vi "Main Page.vi"(8 "error in (no error)":errorcluster, 11 "Node Ptr":T1 format="%.0x") -> (0 "error out":errorcluster)   [LabVIEW 2019, in "Protection and Counter Addon System Explorer.lvlib"]
uses:
  Protection and Counter Addon System Explorer.lvlib
  <vilib>/NI VeriStand/Custom Device API/Custom Device Item Ref.ctl
  <vilib>/NI/NI VeriStand Hardware Resource Discovery/_Types/Filter Type.ctl
  Addon Shared/Types/986x.ctl
  Addon Shared/SubVIs/GUID Lookup.vi
  <vilib>/NI VeriStand/Custom Device API/NI VeriStand - Get Item Property.vi
  <vilib>/NI VeriStand/Custom Device API/Get Item Property (Boolean).vi
  <vilib>/NI VeriStand/Custom Device API/Get Item Property (String).vi
  <vilib>/NI VeriStand/Custom Device API/Get Item Property (Dependent File).vi
  <vilib>/NI VeriStand/Custom Device API/Custom Device API.lvlib
  <vilib>/NI/NI VeriStand Hardware Resource Discovery/NIVS Hardware Discovery.lvlib
  Addon Shared/Protection and Counter Addon Shared.lvlib
panel:
  out "Version":string
  in  "FPGA Settings":cluster{"Section Name":string}={"Section Name"="FPGA Settings"}
  in  "RIO Browse":bool
  in  "RIO Device":string
  in  "Enable Bitfile":bool
  in  "Bitfile Path":path
  in  "Use Legacy":bool
  in  "Loop Priority":i32=100 format="%.0p"
  in  "FD Baud rate [Bd]":u64 format="%.0p"
  in  "CAN I/O Mode":u32(ring) items=["CAN 2.0", "CAN FD", "CAN FD+BRS"]
  in  "Database Settings":cluster{"Section Name":string}={"Section Name"="Database Settings"}
  in  "CAN Browse":bool
  in  "Termination":enum16{"Off", "On"}(ring)
  in  "CAN Port":string
  in  "Baud rate [Bd]":u64 format="%.0p"
  out "XNET Cluster":refnum<k21>
  out "XNET Database":refnum<k21>
  in  "SHDocVw.IWebBrowser2":refnum<k7>(container)
  in  "Header":cluster{"Section Name":string}={"Section Name"="CAN Settings"}
  in  "Name":string
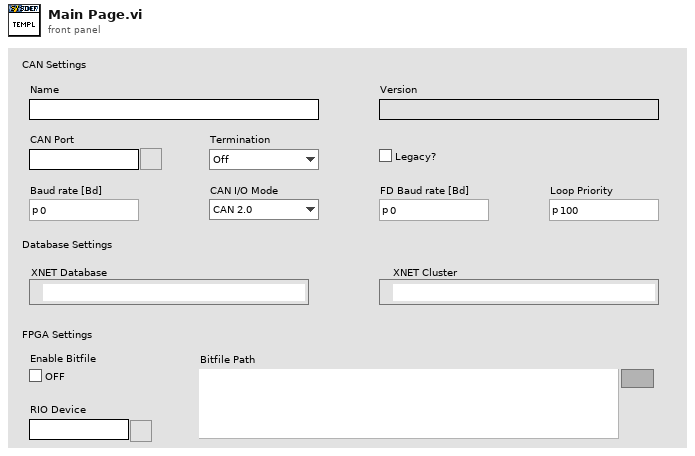
[diagram p1: front panel]
types:
  T1 = typedef "Custom Device API.lvlib/Custom Device Item Ref.ctl" = u64
  T2 = typedef "Protection and Counter Addon Shared.lvlib/986x.ctl" = cluster{"Enable":bool, "RIO Device":string, "Bitfile":path}
  T3 = typedef "Protection and Counter Addon Shared.lvlib/XNET Settings.ctl" = cluster{"Database":refnum<k21>, "Cluster":refnum<k21>, "Port":string, "Baud rate [Bd]":u64, "Termination":u32, "CAN I/O Mode":u32, "FD Baud rate [Bd]":u64, "Priority":i32, "Use Legacy":bool}
  T4 = typedef "Custom Device API.lvlib/Custom Device Item Info.ctl" = cluster{"Name":string, "Is Channel":bool, "GUID":string, "Is Waveform":bool}
  T5 = typedef "NIVS Hardware Discovery.lvlib/Filter Type.ctl" = enum16{"Device Category", "Product Name", "Ethernet", "XNET", "VISA", "FPGA", "EtherCAT Master", "DAQmx", "GPIB", "Serial"}
  T6 = typedef "Custom Device API.lvlib/Custom Device Commands.ctl" = enum16{"Default", "Item renamed", "Shutdown", "Dynamic button pressed"}
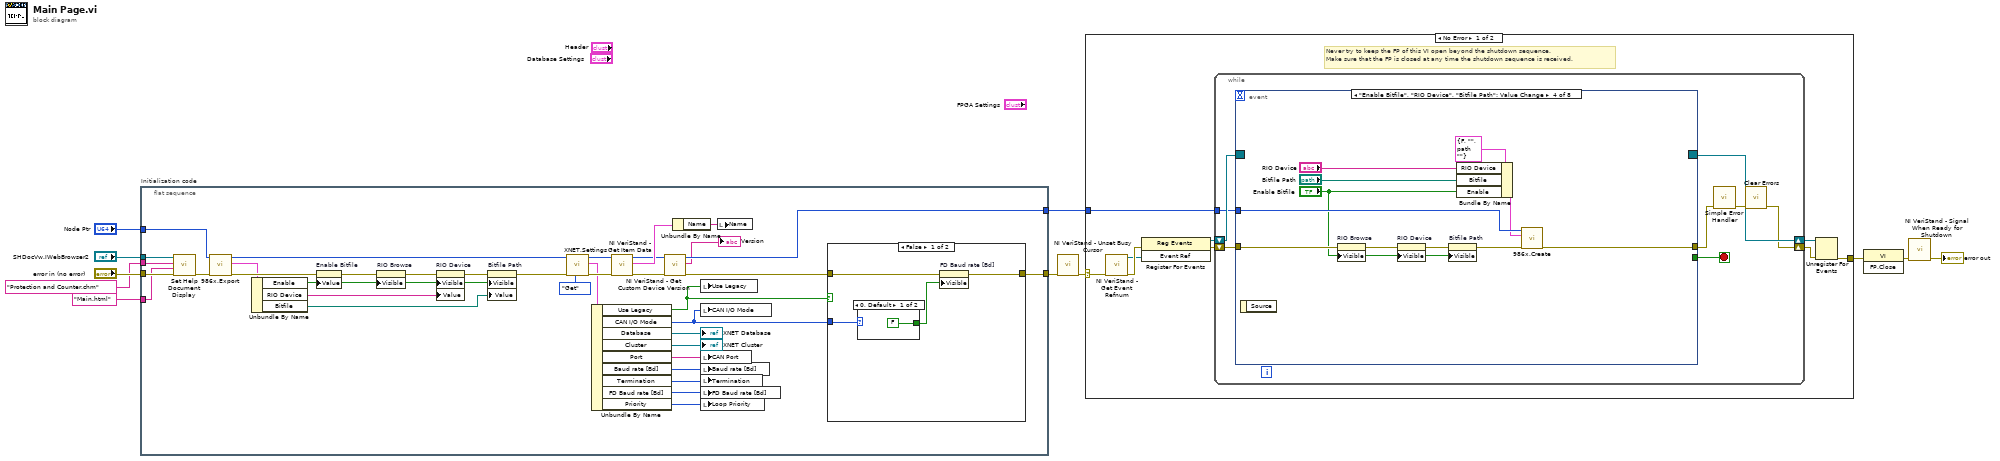
[diagram p0: block diagram]
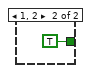
[diagram p2: hidden frame]
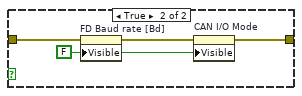
[diagram p3: hidden frame]
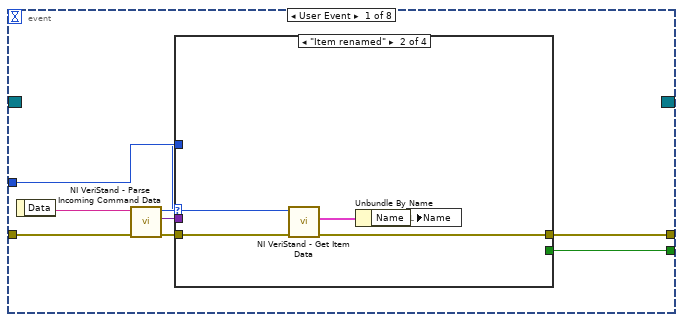
[diagram p4: hidden frame]
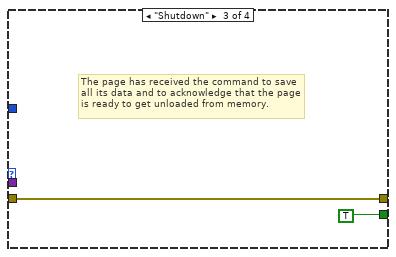
[diagram p6: hidden frame]
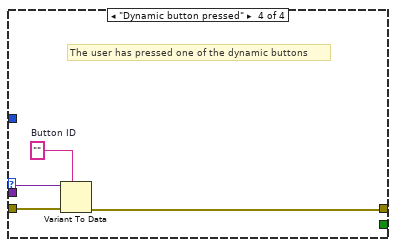
[diagram p7: hidden frame]
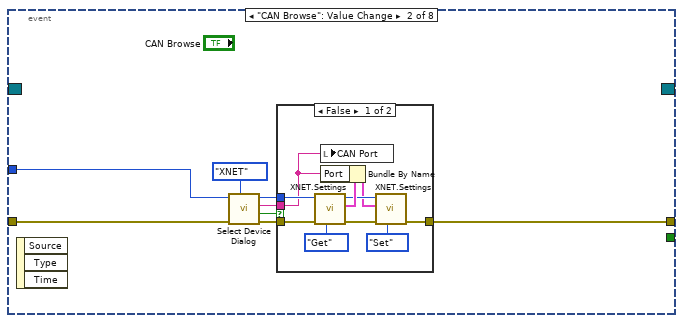
[diagram p8: hidden frame]
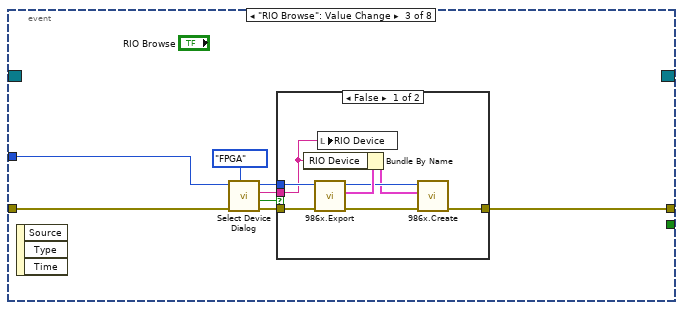
[diagram p10: hidden frame]
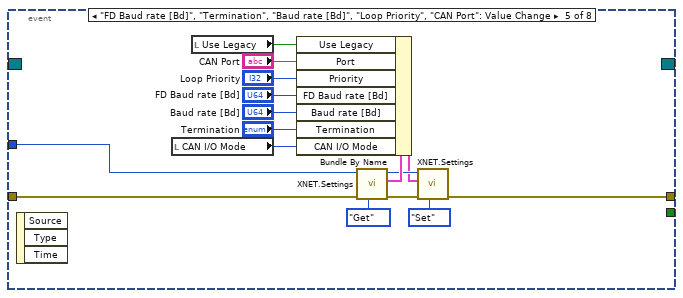
[diagram p12: hidden frame]
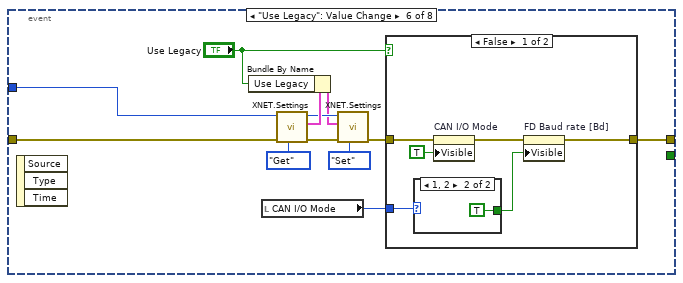
[diagram p13: hidden frame]
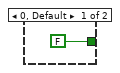
[diagram p14: hidden frame]
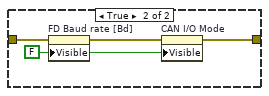
[diagram p15: hidden frame]
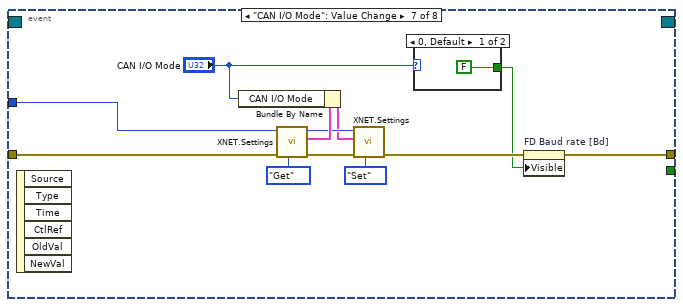
[diagram p16: hidden frame]
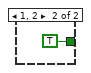
[diagram p17: hidden frame]
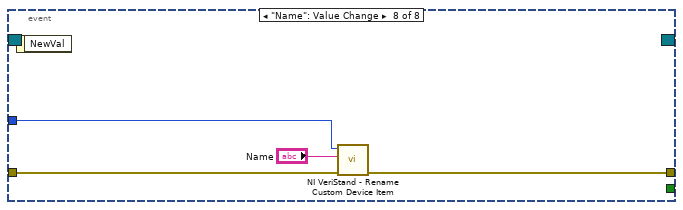
[diagram p18: hidden frame]
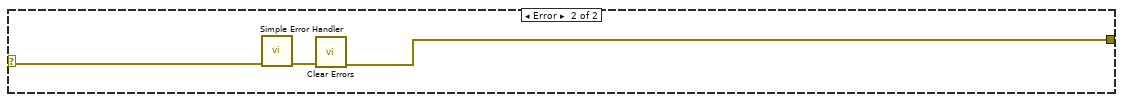
[diagram p19: hidden frame]
diagram:
  n1 = flat-sequence "Initialization code" {
    tunnel: "error in (no error)" -> [w46]
    tunnel: "Node Ptr" -> [w27]
    tunnel: [w30] -> w7
    tunnel: [w13] -> w4
    tunnel: "SHDocVw.IWebBrowser2" -> [w45]
    tunnel: "Protection and Counter.chm" ("Main CHM File") -> [w44]
    tunnel: "Main.html" ("HTML File") -> [w43]
    frame #0 {
      n2 = call "Set Help Document Display.vi"("error in (no error)"=w46, "HTML File"=w43, "Main CHM File"=w44, "SHDocVw.IWebBrowser2"=w45) -> ("error out"=w28:errorcluster)  [unwired: 7 in]
      n3 = call "986x.Export.vi"("error in (no error)"=w28, "Device Item Ref in"=w27) -> ("error out"=w22:errorcluster, "986x Support"=w20:T2, "Item Ref out"=w26:T1)  [unwired: 7 in]
      n4 = Unbundle By Name(w20) -> ("Enable"=w19:bool, "RIO Device"=w18:string, "Bitfile"=w17:path)
      n5 = property on="Enable Bitfile" class="Bool (strict)"(error in=w22, "Value"=w19) -> (error out=w25:errorcluster)  [unwired: 1 in, 1 out]
      n6 = property on="RIO Browse" class="Bool"(error in=w25, "Visible"=w19) -> (error out=w24:errorcluster)  [unwired: 1 in, 1 out]
      n7 = property on="RIO Device" class="Str"(error in=w24, "Visible"=w19, "Value"=w18) -> (error out=w23:errorcluster)  [unwired: 1 in, 1 out]
      n8 = property on="Bitfile Path" class="Path"(error in=w23, "Visible"=w19, "Value"=w17) -> (error out=w21:errorcluster)  [unwired: 1 in, 1 out]
      n9 = call "XNET.Settings.vi"("Action"=enum8{"Get", "Set"}."Get", "error in (no error)"=w21, "Parent Ref in"=w26) -> ("error out"=w42:errorcluster, "XNET Settings"=w39:T3, "Item Ref out"=w41:T1)  [unwired: 6 in]
      n10 = Unbundle By Name(w39) -> ("Use Legacy"=w31:bool, "CAN I/O Mode"=w29:u32, "Database"=→"XNET Database":refnum<k21>, "Cluster"=→"XNET Cluster":refnum<k21>, "Port"=w36:string, "Baud rate [Bd]"=w35:u64, "Termination"=w34:u32, "FD Baud rate [Bd]"=w33:u64, "Priority"=w32:i32)
      n11 = call <vilib>:"NI VeriStand - Get Item Data.vi"("error in (no error)"=w42, "Item Ref in"=w41) -> ("error out"=w16:errorcluster, "Item Info"=w48:T4, "Item Ref out"=w14:T1)  [unwired: 7 out]
      n12 = call <vilib>:"NI VeriStand - Get Custom Device Version.vi"("error in (no error)"=w16, "Device Ref in"=w14) -> ("error out"=w15:errorcluster, "Value"=→"Version":string, "Device Ref out"=w13:T1)  [unwired: 7 in]
      n13 = Unbundle By Name(w48) -> ("Name"=w47:string)
      n14 = local write "Use Legacy"(w31) -> ()
      n15 = local write "CAN I/O Mode"(w29) -> ()
      n16 = local write "CAN Port"(w36) -> ()
      n17 = local write "Baud rate [Bd]"(w35) -> ()
      n18 = local write "Termination"(w34) -> ()
      n19 = local write "FD Baud rate [Bd]"(w33) -> ()
      n20 = local write "Loop Priority"(w32) -> ()
      n21 = local write "Name"(w47) -> ()
      n22 = case shown="False" w31 {
        tunnel: w15 -> [w51 w57]
        tunnel: [w50 w56] -> w30
        tunnel: w29 -> [w52 _]
        frame False {
          n23 = case shown="0, Default" w52 {
            tunnel: [FALSE TRUE] -> w49
            frame 0, Default {
            }
            frame 1, 2 {
            }
          }
          n24 = property on="FD Baud rate [Bd]" class="DigNum (strict)"(error in=w51, "Visible"=w49) -> (error out=w50:errorcluster)  [unwired: 1 in, 1 out]
        }
        frame True {
          w55 = FALSE ("Visible")
          n25 = property on="FD Baud rate [Bd]" class="DigNum (strict)"(error in=w57, "Visible"=w55) -> (error out=w58:errorcluster)  [unwired: 1 in, 1 out]
          n26 = property on="CAN I/O Mode" class="Ring (strict)"(error in=w58, "Visible"=w55) -> (error out=w56:errorcluster)  [unwired: 1 in, 1 out]
        }
      }
    }
  }
  n27 = call <vilib>:"NI VeriStand - Unset Busy Cursor.vi"("error in (no error)"=w7) -> ("error out"=w6:errorcluster)  [unwired: 10 out]
  n28 = case shown="No Error" w6 {
    selector: w6 -> [w59 w203]
    tunnel: [w64 w201] -> w11
    tunnel: w4 -> [w60 _]
    frame No Error {
      # "Never try to keep the FP of this VI open beyond the shutdown sequence.\nMake sure that the FP is closed at any time the shutdown sequence is received."
      n29 = call <vilib>:"NI VeriStand - Get Event Refnum.vi"("error in (no error)"=w59) -> ("error out"=w67:errorcluster, "Event Ref"=w63:refnum<user-event>)  [unwired: 9 out]
      n30 = register-events(error in=w67, w63) -> (reference out=w61:refnum<event-registration>, error out=w62:errorcluster)  [unwired: 1 in]
      n31 = while {
        tunnel: w60 -> [w71]
        shift-right: [w68] -> w65
        shift-left: w62 -> [w74]
        shift-right: [w75] -> w66
        shift-left: w61 -> [w73]
        stop <- w72 stop-if-true
        n32 = event shown="[3] \"Enable Bitfile\", \"RIO Device\", \"Bitfile Path\": Value Change" {
          selector: w73 -> [_ _ _ _ _ _ _ _]
          dyn-events: [_ _ _ _ _ _ _ _] -> w75
          timeout: _ -> [_ _ _ _ _ _ _ _]
          tunnel: w74 -> [w83 w98 w117 w139 w152 w164 w188 w200]
          tunnel: [w79 _ _ _ _ _ _ _] -> w72
          tunnel: [w78 w96 w115 w142 w151 w160 w185 w199] -> w70
          tunnel: w71 -> [w77 w97 w116 w137 w150 w163 w187 w198]
          event User Event {
            n33 = event-data() -> ("Data"=w82:string)  [unwired: 1 out]
            n34 = call <vilib>:"NI VeriStand - Parse Incoming Command Data.vi"("error in (no error)"=w83, "Incoming data"=w82) -> ("error out"=w81:errorcluster, "Outgoing data"=w76:variant, "Action"=w80:T6)  [unwired: 7 out]
            n35 = case shown="\"Item renamed\"" w80 {
              tunnel: w81 -> [w84 w89 w90 w95]
              tunnel: [_ _ TRUE _] -> w79
              tunnel: [w84 w86 w90 w92] -> w78
              tunnel: w77 -> [_ w88 _ _]
              tunnel: w76 -> [_ _ _ w94]
              frame "Default", Default {
              }
              frame "Item renamed" {
                n36 = call <vilib>:"NI VeriStand - Get Item Data.vi"("error in (no error)"=w89, "Item Ref in"=w88) -> ("error out"=w86:errorcluster, "Item Info"=w87:T4)  [unwired: 8 out]
                n37 = Unbundle By Name(w87) -> ("Name"=w85:string)
                n38 = local write "Name"(w85) -> ()
              }
              frame "Shutdown" {
                # "The page has received the command to save all its data and to acknowledge that the page is ready to get unloaded from memory."
              }
              frame "Dynamic button pressed" {
                w93 = ""  # Button ID
                # "The user has pressed one of the dynamic buttons"
                n39 = Variant To Data(error in=w95, type=w93, Variant=w94) -> (error out=w92:errorcluster)  [unwired: 1 out]
              }
            }
          }
          event "CAN Browse": Value Change {
            n40 = event-data() -> ()  [unwired: 4 out]
            n41 = call <vilib>:"Select Device Dialog.vi"("Filter Type"=Filter_Type."XNET", "error in (no error)"=w98, "Item Ref in"=w97) -> ("error out"=w102:errorcluster, "Cancelled?"=w101:bool, "Selected Alias"=w100:string, "Item Ref out"=w103:T1)  [unwired: 5 in]
            n42 = case shown="False" w101 {
              tunnel: w103 -> [w111 _]
              tunnel: [w108 w114] -> w96
              tunnel: w102 -> [w105 w114]
              tunnel: w100 -> [w104 _]
              frame False {
                n43 = call "XNET.Settings.vi"("Action"=enum8{"Get", "Set"}."Get", "error in (no error)"=w105, "Parent Ref in"=w111) -> ("error out"=w106:errorcluster, "XNET Settings"=w112:T3, "Item Ref out"=w109:T1)  [unwired: 6 in]
                n44 = local write "CAN Port"(w104) -> ()
                n45 = Bundle By Name(cluster=w112, "Port"=w104) -> (w107:T3)
                n46 = call "XNET.Settings.vi"("Action"=enum8{"Get", "Set"}."Set", "error in (no error)"=w106, "XNET Settings"=w107, "Parent Ref in"=w109) -> ("error out"=w108:errorcluster)  [unwired: 5 in, 2 out]
              }
              frame True {
              }
            }
          }
          event "RIO Browse": Value Change {
            n47 = event-data() -> ()  [unwired: 4 out]
            n48 = call <vilib>:"Select Device Dialog.vi"("Filter Type"=Filter_Type."FPGA", "error in (no error)"=w117, "Item Ref in"=w116) -> ("error out"=w121:errorcluster, "Cancelled?"=w120:bool, "Selected Alias"=w119:string, "Item Ref out"=w122:T1)  [unwired: 5 in]
            n49 = case shown="False" w120 {
              tunnel: w122 -> [w129 _]
              tunnel: [w124 w131] -> w115
              tunnel: w121 -> [w128 w131]
              tunnel: w119 -> [w127 _]
              frame False {
                n50 = call "986x.Export.vi"("error in (no error)"=w128, "Device Item Ref in"=w129) -> ("error out"=w126:errorcluster, "986x Support"=w130:T2, "Item Ref out"=w125:T1)  [unwired: 7 in]
                n51 = Bundle By Name(cluster=w130, "RIO Device"=w127) -> (w123:T2)
                n52 = local write "RIO Device"(w127) -> ()
                n53 = call "986x.Create.vi"("error in (no error)"=w126, "986x Support"=w123, "Device Item Ref in"=w125) -> ("error out"=w124:errorcluster)  [unwired: 7 in, 1 out]
              }
              frame True {
              }
            }
          }
          event "Enable Bitfile", "RIO Device", "Bitfile Path": Value Change {
            n54 = event-data() -> ()  [unwired: 2 out]
            n55 = property on="RIO Browse" class="Bool"(error in=w139, "Visible"="Enable Bitfile") -> (error out=w140:errorcluster)  [unwired: 1 in, 1 out]
            n56 = property on="RIO Device" class="Str"(error in=w140, "Visible"="Enable Bitfile") -> (error out=w141:errorcluster)  [unwired: 1 in, 1 out]
            n57 = property on="Bitfile Path" class="Path"(error in=w141, "Visible"="Enable Bitfile") -> (error out=w138:errorcluster)  [unwired: 1 in, 1 out]
            n58 = Bundle By Name(cluster=T2 {"Enable"=FALSE, "RIO Device"="", "Bitfile"=path ""} ("986x Support"), "RIO Device"="RIO Device", "Bitfile"="Bitfile Path", "Enable"="Enable Bitfile") -> (w135:T2)
            n59 = call "986x.Create.vi"("error in (no error)"=w138, "986x Support"=w135, "Device Item Ref in"=w137) -> ("error out"=w142:errorcluster)  [unwired: 7 in, 1 out]
          }
          event "FD Baud rate [Bd]", "Termination", "Baud rate [Bd]", "Loop Priority", "CAN Port": Value Change {
            n60 = event-data() -> ()  [unwired: 4 out]
            n61 = local read "CAN I/O Mode"() -> (w143:u32)
            n62 = local read "Use Legacy"() -> (w144:bool)
            n63 = call "XNET.Settings.vi"("Action"=enum8{"Get", "Set"}."Get", "error in (no error)"=w152, "Parent Ref in"=w150) -> ("error out"=w153:errorcluster, "XNET Settings"=w157:T3, "Item Ref out"=w155:T1)  [unwired: 6 in]
            n64 = Bundle By Name(cluster=w157, "Use Legacy"=w144, "Port"="CAN Port", "Priority"="Loop Priority", "FD Baud rate [Bd]"="FD Baud rate [Bd]", "Baud rate [Bd]"="Baud rate [Bd]", "Termination"="Termination", "CAN I/O Mode"=w143) -> (w154:T3)
            n65 = call "XNET.Settings.vi"("Action"=enum8{"Get", "Set"}."Set", "error in (no error)"=w153, "XNET Settings"=w154, "Parent Ref in"=w155) -> ("error out"=w151:errorcluster)  [unwired: 5 in, 2 out]
          }
          event "Use Legacy": Value Change {
            n66 = event-data() -> ()  [unwired: 4 out]
            n67 = local read "CAN I/O Mode"() -> (w159:u32)
            n68 = call "XNET.Settings.vi"("Action"=enum8{"Get", "Set"}."Get", "error in (no error)"=w164, "Parent Ref in"=w163) -> ("error out"=w165:errorcluster, "XNET Settings"=w169:T3, "Item Ref out"=w167:T1)  [unwired: 6 in]
            n69 = Bundle By Name(cluster=w169, "Use Legacy"="Use Legacy") -> (w166:T3)
            n70 = call "XNET.Settings.vi"("Action"=enum8{"Get", "Set"}."Set", "error in (no error)"=w165, "XNET Settings"=w166, "Parent Ref in"=w167) -> ("error out"=w161:errorcluster)  [unwired: 5 in, 2 out]
            n71 = case shown="False" "Use Legacy" {
              tunnel: w161 -> [w173 w181]
              tunnel: [w176 w180] -> w160
              tunnel: w159 -> [w174 _]
              frame False {
                n72 = case shown="1, 2" w174 {
                  tunnel: [FALSE TRUE] -> w175
                  frame 0, Default {
                  }
                  frame 1, 2 {
                  }
                }
                n73 = property on="CAN I/O Mode" class="Ring (strict)"(error in=w173, "Visible"=TRUE) -> (error out=w172:errorcluster)  [unwired: 1 in, 1 out]
                n74 = property on="FD Baud rate [Bd]" class="DigNum (strict)"(error in=w172, "Visible"=w175) -> (error out=w176:errorcluster)  [unwired: 1 in, 1 out]
              }
              frame True {
                w179 = FALSE ("Visible")
                n75 = property on="FD Baud rate [Bd]" class="DigNum (strict)"(error in=w181, "Visible"=w179) -> (error out=w182:errorcluster)  [unwired: 1 in, 1 out]
                n76 = property on="CAN I/O Mode" class="Ring (strict)"(error in=w182, "Visible"=w179) -> (error out=w180:errorcluster)  [unwired: 1 in, 1 out]
              }
            }
          }
          event "CAN I/O Mode": Value Change {
            n77 = event-data() -> ()  [unwired: 7 out]
            n78 = call "XNET.Settings.vi"("Action"=enum8{"Get", "Set"}."Get", "error in (no error)"=w188, "Parent Ref in"=w187) -> ("error out"=w189:errorcluster, "XNET Settings"=w193:T3, "Item Ref out"=w191:T1)  [unwired: 6 in]
            n79 = Bundle By Name(cluster=w193, "CAN I/O Mode"="CAN I/O Mode") -> (w190:T3)
            n80 = call "XNET.Settings.vi"("Action"=enum8{"Get", "Set"}."Set", "error in (no error)"=w189, "XNET Settings"=w190, "Parent Ref in"=w191) -> ("error out"=w186:errorcluster)  [unwired: 5 in, 2 out]
            n81 = case shown="0, Default" "CAN I/O Mode" {
              tunnel: [FALSE TRUE] -> w184
              frame 0, Default {
              }
              frame 1, 2 {
              }
            }
            n82 = property on="FD Baud rate [Bd]" class="DigNum (strict)"(error in=w186, "Visible"=w184) -> (error out=w185:errorcluster)  [unwired: 1 in, 1 out]
          }
          event "Name": Value Change {
            n83 = event-data() -> ()  [unwired: 2 out]
            n84 = call <vilib>:"NI VeriStand - Rename Custom Device Item.vi"("error in (no error)"=w200, "New Name"="Name", "Item Ref in"=w198) -> ("error out"=w199:errorcluster)  [unwired: 1 in, 7 out]
          }
        }
        n85 = call <vilib>:"Simple Error Handler.vi"("error in (no error)"=w70) -> ("error out"=w69:errorcluster)  [unwired: 1 in, 7 out]
        n86 = call <vilib>:"Clear Errors.vi"("error in (no error)"=w69) -> ("error out"=w68:errorcluster)  [unwired: 1 in, 5 out]
      }
      n87 = Unregister For Events(event registration refnum=w66, error in=w65) -> (error out=w64:errorcluster)
    }
    frame Error {
      n88 = call <vilib>:"Simple Error Handler.vi"("error in (no error)"=w203) -> ("error out"=w202:errorcluster)  [unwired: 1 in, 7 out]
      n89 = call <vilib>:"Clear Errors.vi"("error in (no error)"=w202) -> ("error out"=w201:errorcluster)  [unwired: 1 in, 5 out]
    }
  }
  n90 = invoke class="VI" method="FP.Close"(error in=w11) -> (error out=w10:errorcluster)  [unwired: 2 in, 2 out]
  n91 = call <vilib>:"NI VeriStand - Signal When Ready for Shutdown.vi"("error in (no error)"=w10) -> ("error out"=→"error out":errorcluster)  [unwired: 10 out]
